vi "ConnectionDataRead.vi"(8 "error in (no error)":errorcluster, 9 "ReadData":refnum<class "ReadData.lvclass">, 10 "Connection":refnum<class "Connection.lvclass">, 11 "TcpServer in":refnum<class "TcpServer.lvclass">) -> (0 "error out":errorcluster, 3 "TcpServer out":refnum<class "TcpServer.lvclass">)   [LabVIEW 2022 SP3, in "TcpServer.lvlib" / "TcpServer.lvclass"]
uses:
  TcpServer.lvclass
  C:/Program Files (x86)/National Instruments/LabVIEW 2022/vi.lib/ActorFramework/Actor/Actor.lvclass
  C:/Users/jakub/repos/gh/sw4sys/lv-tcp-server-sample/LoggingActor/Source/LoggingActor/LoggingActor/LoggingActor.lvclass
  TcpSocket/Source/TcpSocket/Connection/Connection.lvclass
  Connection/ReadData/ReadData.lvclass
  <vilib>/ActorFramework/Actor/Actor.lvclass/Actor.ctl
  TcpServer.lvclass/TcpServer.ctl
  Connection/ReadData/ReadData.lvclass/ReadData.ctl
  TcpSocket/Source/TcpSocket/Connection/Connection.lvclass/Connection.ctl
  LoggingActor/Source/LoggingActor/LoggingActor/LoggingActor.lvclass/LoggingActor.ctl
  CallerMessage Messages/TcpDataReceived Msg/TcpDataReceived Msg.lvclass/TcpDataReceived Msg.ctl
  <vilib>/ActorFramework/Message Enqueuer/Message Enqueuer.lvclass/Message Enqueuer.ctl
  LoggingActor/Source/LoggingActor/LoggingActor/Read Logger.vi
  TcpSocket/Source/TcpSocket/Connection/Read Address.vi
  TcpSocket/Source/TcpSocket/Connection/Read Port.vi
  TcpSocket/Source/TcpSocket/Connection/Read Connection.vi
  TcpSocket/Source/TcpSocket/Connection/Read ReadMode.vi
  TcpSocket/Source/TcpSocket/Connection/Read ReadTimeout.vi
  TcpSocket/Source/TcpSocket/Connection/Read WriteTimeout.vi
  Connection/ReadData/Read Data.vi
  Connection/ReadData/Read TimeStamp.vi
  Connection/ReadData/Read ReadNumber.vi
  <vilib>/ActorFramework/Message Enqueuer/Enqueue.vi
  CallerMessage Messages/TcpDataReceived Msg/TcpDataReceived Msg.lvclass
  C:/Program Files (x86)/National Instruments/LabVIEW 2022/vi.lib/ActorFramework/Message/Message.lvclass
  <vilib>/ActorFramework/Message Priority Queue/Priority Enqueue.vi
  <vilib>/ActorFramework/Message Enqueuer/Message Enqueuer.lvclass
  Logger/Source/Logger/Logger.lvclass
  DataReceived/DataReceived.lvclass
  <vilib>/ActorFramework/Actor/Actor.lvclass
  StringUtils/Source/StringUtils/StringUtils.lvlib
  C:/Users/jakub/repos/gh/sw4sys/lv-tcp-server-sample/TcpServerSample/Source/TcpServerSample/TcpServer/TcpServer/TcpServer.lvclass
  C:/Users/jakub/repos/gh/sw4sys/lv-tcp-server-sample/TcpServerSample/Source/TcpServerSample/Connection/CallerMessage/CallerMessage.lvclass
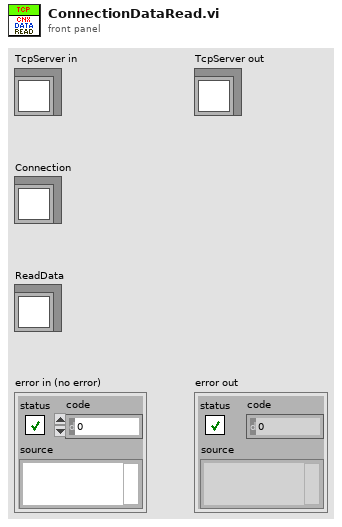
[diagram p1: front panel]
types:
  T1 = enum16{"Standard", "Buffered", "CRLF", "Immediate"}
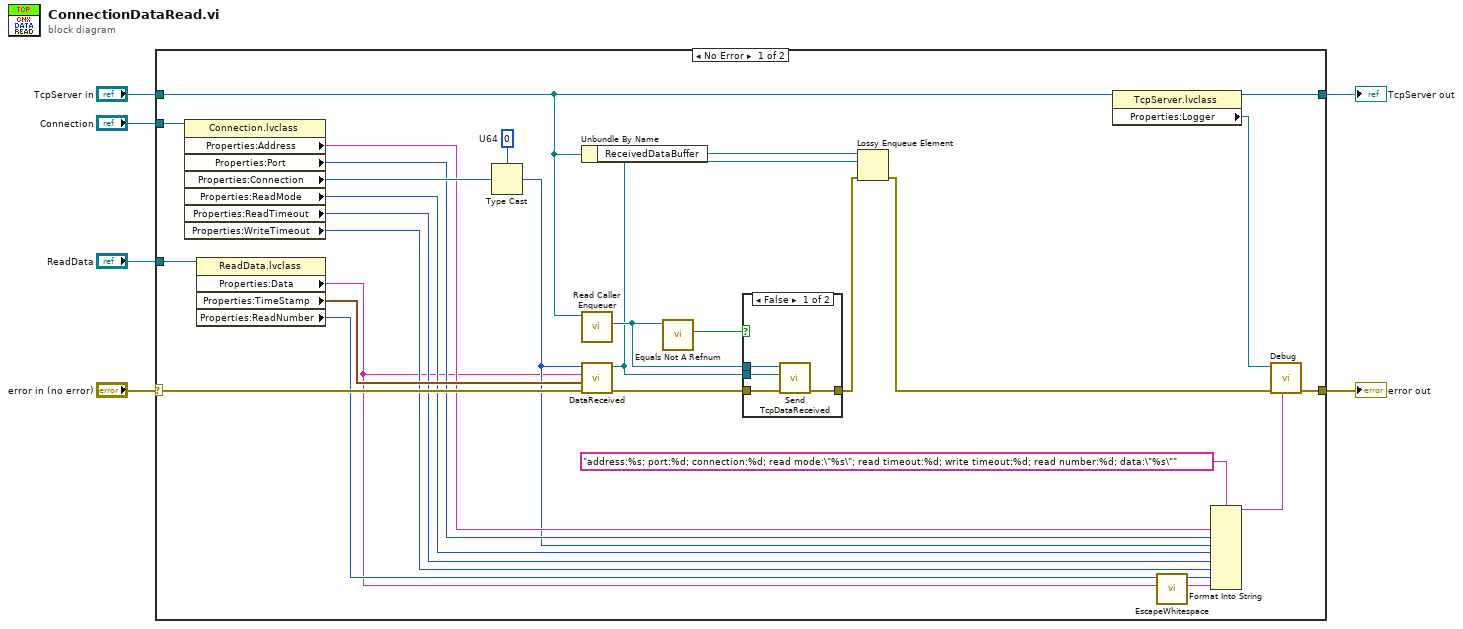
[diagram p0: block diagram]
diagram:
  n1 = case shown="No Error" "error in (no error)" {
    selector: "error in (no error)" -> [w29 w41]
    tunnel: "ReadData" -> [w34 _]
    tunnel: "Connection" -> [w22 _]
    tunnel: [w25 w41] -> w4
    tunnel: "TcpServer in" -> [w10 w40]
    tunnel: [w26 w40] -> w1
    frame No Error {
      w32 = u64 0  # U64
      n2 = property class="Connection.lvclass"(reference=w22) -> ("Properties:Address"=w21:string, "Properties:Port"=w20:u16, "Properties:Connection"=w33:refnum<k5>, "Properties:ReadMode"=w18:T1, "Properties:ReadTimeout"=w17:i32, "Properties:WriteTimeout"=w16:i32)  [unwired: 1 in, 2 out]
      n3 = property class="ReadData.lvclass"(reference=w34) -> ("Properties:Data"=w14:string, "Properties:TimeStamp"=w31:timestamp, "Properties:ReadNumber"=w15:u32)  [unwired: 1 in, 2 out]
      n4 = Type Cast(type=w32, x=w33) -> (*(type *) &x=w19:u64)
      n5 = Unbundle By Name(w10) -> ("ReceivedDataBuffer"=w9:refnum<queue>)
      n6 = call <vilib>:"Read Caller Enqueuer.vi"("Actor"=w10) -> ("Caller Enqueuer"=w28:refnum<class "Message Enqueuer.lvclass">)  [unwired: 10 in]
      n7 = call "DataReceived.vi"("error in (no error)"=w29, "TimeStamp"=w31, "Data"=w14, "Refnum"=w19) -> ("error out"=w30:errorcluster, "DataReceived"=w11:refnum<class "DataReceived.lvclass">)  [unwired: 6 in]
      n8 = call <vilib>:"Equals Not A Refnum.vi"("Message Enqueuer"=w28) -> ("Not a refnum?"=w27:bool)  [unwired: 10 in]
      n9 = case shown="False" w27 {
        tunnel: w30 -> [w38 w39]
        tunnel: [w37 w39] -> w8
        tunnel: w11 -> [w36 _]
        tunnel: w28 -> [w35 _]
        frame False {
          n10 = call "Send TcpDataReceived.vi"("error in (no error)"=w38, "DataReceived"=w36, "Message Enqueuer"=w35) -> ("error out"=w37:errorcluster)  [unwired: 7 in, 1 out]
        }
        frame True {
        }
      }
      n11 = Lossy Enqueue Element(queue=w9, element=w11, error in (no error)=w8) -> (error out=w7:errorcluster)  [unwired: 3 out]
      n12 = property class="TcpServer.lvclass"(reference=w10) -> (reference out=w26:refnum<class "TcpServer.lvclass">, "Properties:Logger"=w24:refnum<class "Logger.lvclass">)  [unwired: 1 in, 1 out]
      n13 = call "EscapeWhitespace.vi"("InputString"=w14) -> ("EscapedWhitespace"=w13:string)  [unwired: 10 in]
      n14 = Format Into String(format string="address:%s; port:%d; connection:%d; read mode:\"%s\"; read timeout:%d; write timeout:%d; read number:%d; data:\"%s\"", w21, w20, w19, w18, w17, w16, w15, w13) -> (resulting string=w12:string)  [unwired: 2 in, 1 out]
      n15 = call-dynamic "Debug.vi"("Message"=w12, "error in (no error)"=w7, "Logger in"=w24) -> ("error out"=w25:errorcluster)  [unwired: 5 in, 1 out]
    }
    frame Error {
    }
  }
  "error out" <- w4
  "TcpServer out" <- w1
